vi "axc license check out.vi"(8 "error in (no error)":errorcluster caption="错误输入（无错误）") -> (0 "error out":errorcluster caption="错误输出")   [LabVIEW 2015, in "asf_lic.lvlib"]
doc: "AX_LIC_EXPORTS void axc_license_check_out();"
uses:
  asf_lic.lvlib
  asf_lic.dll
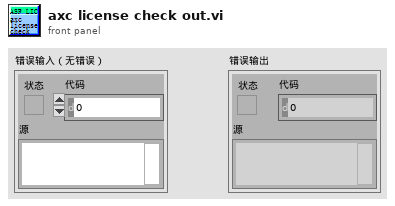
[diagram p1: front panel]
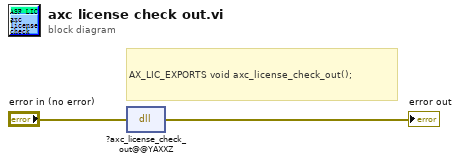
[diagram p0: block diagram]
diagram:
  # "AX_LIC_EXPORTS void axc_license_check_out();"
  n1 = dll-call lib="PTH2>abs CUsersSpesTechDesktopdist-lic函数\tasf_lic.*" fn="?axc_license_check_out@@YAXXZ"(error in="error in (no error)") -> (error out=→"error out":errorcluster)  [unwired: 3 in, 1 out]
